vi "ECG_YY.vi"() -> ()   [LabVIEW 2020]
uses:
  <vilib>/Analysis/3filter.llb/Filter Passband Type.ctl
  <vilib>/Analysis/2dsp.llb/Real FFT.vi
  <vilib>/Utility/file.llb/Read Delimited Spreadsheet (DBL).vi
  <vilib>/Analysis/3filter.llb/Butterworth Filter (DBL).vi
  <vilib>/Analysis/NI_AALBase.lvlib
  <vilib>/Analysis/NI_AALPro.lvlib
panel:
  out "YY_stimuli4":dbl[](graph)
  out "YY_stimuli3":dbl[](graph)
  out "YY_stimuli1":dbl[](graph)
  out "YY_baseline":dbl[](graph)
  out "YY_stimuli 2":dbl[](graph)
  out "RRI_series_YY_baseline 2":dbl[](graph)
  out "PS_YY_stimuli4":cluster{"x":dbl, "x":dbl, dbl[]}(graph)
  out "PS_YY_stimuli 2":cluster{"x":dbl, "x":dbl, dbl[]}(graph)
  out "PS_YY_stimuli3":cluster{"x":dbl, "x":dbl, dbl[]}(graph)
  out "PS_YY_stimuli1":cluster{"x":dbl, "x":dbl, dbl[]}(graph)
  out "PS_YY_baseline":cluster{"x":dbl, "x":dbl, dbl[]}(graph)
  out "RRI_series_YY_stimuli4":dbl[](graph)
  out "RRI_series_YY_stimuli3":dbl[](graph)
  out "RRI_series_YY_stimuli2":dbl[](graph)
  out "RRI_series_YY_stimuli1":dbl[](graph)
  out "RRI_series_YY_baseline":dbl[](graph)
  out "YY_stimuli4":dbl[](graph)
  out "YY_stimuli3":dbl[](graph)
  out "YY_stimuli 2":dbl[](graph)
  out "YY_stimuli1":dbl[](graph)
  out "YY_baseline":dbl[](graph)
  out "psd_size 5":i32
  out "PS_WD_stimuli4":cluster{"x":dbl, "x":dbl, dbl[]}(graph)
  out "LF/HF 5":dbl
  out "HF  2":dbl
  out "LF  2":dbl
  out "TP (<=0.4Hz)  2":dbl
  out "RRI_size 5":i32
  out "RRI_series_YY_stimuli4":dbl[](graph)
  out "RRI series 5":dbl[](array[numeric])
  out "size(s) 5":i32
  out "2nd Derivatives 5":dbl[](array[numeric])
  out "Amplitudes 5":dbl[](array[numeric])
  out "amplitude 5":dbl[](array[numeric])
  out "location 5":dbl[](array[numeric])
  out "Locations 5":dbl[](array[numeric])
  in  "file path (dialog if empty) 5":path
  out "psd_size 4":i32
  out "PS_WD_stimuli3":cluster{"x":dbl, "x":dbl, dbl[]}(graph)
  out "LF/HF 4":dbl
  out "HF  2":dbl
  out "LF  2":dbl
  out "TP (<=0.4Hz)  2":dbl
  out "RRI_size 4":i32
  out "RRI_series_YY_stimuli3":dbl[](graph)
  out "RRI series 4":dbl[](array[numeric])
  out "size(s) 4":i32
  out "2nd Derivatives 4":dbl[](array[numeric])
  out "Amplitudes 4":dbl[](array[numeric])
  out "amplitude 4":dbl[](array[numeric])
  out "location 4":dbl[](array[numeric])
  out "Locations 4":dbl[](array[numeric])
  in  "file path (dialog if empty) 4":path
  out "psd_size 3":i32
  out "PS_WD_stimuli 2":cluster{"x":dbl, "x":dbl, dbl[]}(graph)
  out "LF/HF 3":dbl
  out "HF  2":dbl
  out "LF  2":dbl
  out "TP (<=0.4Hz)  2":dbl
  out "RRI_size 3":i32
  out "RRI_series_YY_stimuli2":dbl[](graph)
  out "RRI series 3":dbl[](array[numeric])
  out "size(s) 3":i32
  out "2nd Derivatives 3":dbl[](array[numeric])
  out "Amplitudes 3":dbl[](array[numeric])
  out "amplitude 3":dbl[](array[numeric])
  out "location 3":dbl[](array[numeric])
  out "Locations 3":dbl[](array[numeric])
  in  "file path (dialog if empty) 3":path
  out "psd_size 2":i32
  out "PS_WD_stimuli1":cluster{"x":dbl, "x":dbl, dbl[]}(graph)
  out "LF/HF 2":dbl
  out "HF  2":dbl
  out "LF  2":dbl
  out "TP (<=0.4Hz)  2":dbl
  out "RRI_size 2":i32
  out "RRI_series_YY_stimuli1":dbl[](graph)
  out "RRI series 2":dbl[](array[numeric])
  out "size(s) 2":i32
  out "2nd Derivatives 2":dbl[](array[numeric])
  out "Amplitudes 2":dbl[](array[numeric])
  out "amplitude 2":dbl[](array[numeric])
  out "location 2":dbl[](array[numeric])
  out "Locations 2":dbl[](array[numeric])
  in  "file path (dialog if empty) 2":path
  out "psd_size":i32
  out "PS_WD_baseline":cluster{"x":dbl, "x":dbl, dbl[]}(graph)
  out "LF/HF":dbl
  out "HF":dbl
  out "LF":dbl
  out "TP (<=0.4Hz)":dbl
  out "RRI_size":i32
  out "RRI_series_YY_baseline":dbl[](graph)
  out "RRI series":dbl[](array[numeric])
  out "size(s)":i32
  out "2nd Derivatives":dbl[](array[numeric])
  out "Amplitudes":dbl[](array[numeric])
  out "amplitude":dbl[](array[numeric])
  out "location":dbl[](array[numeric])
  out "Locations":dbl[](array[numeric])
  in  "file path (dialog if empty)":path
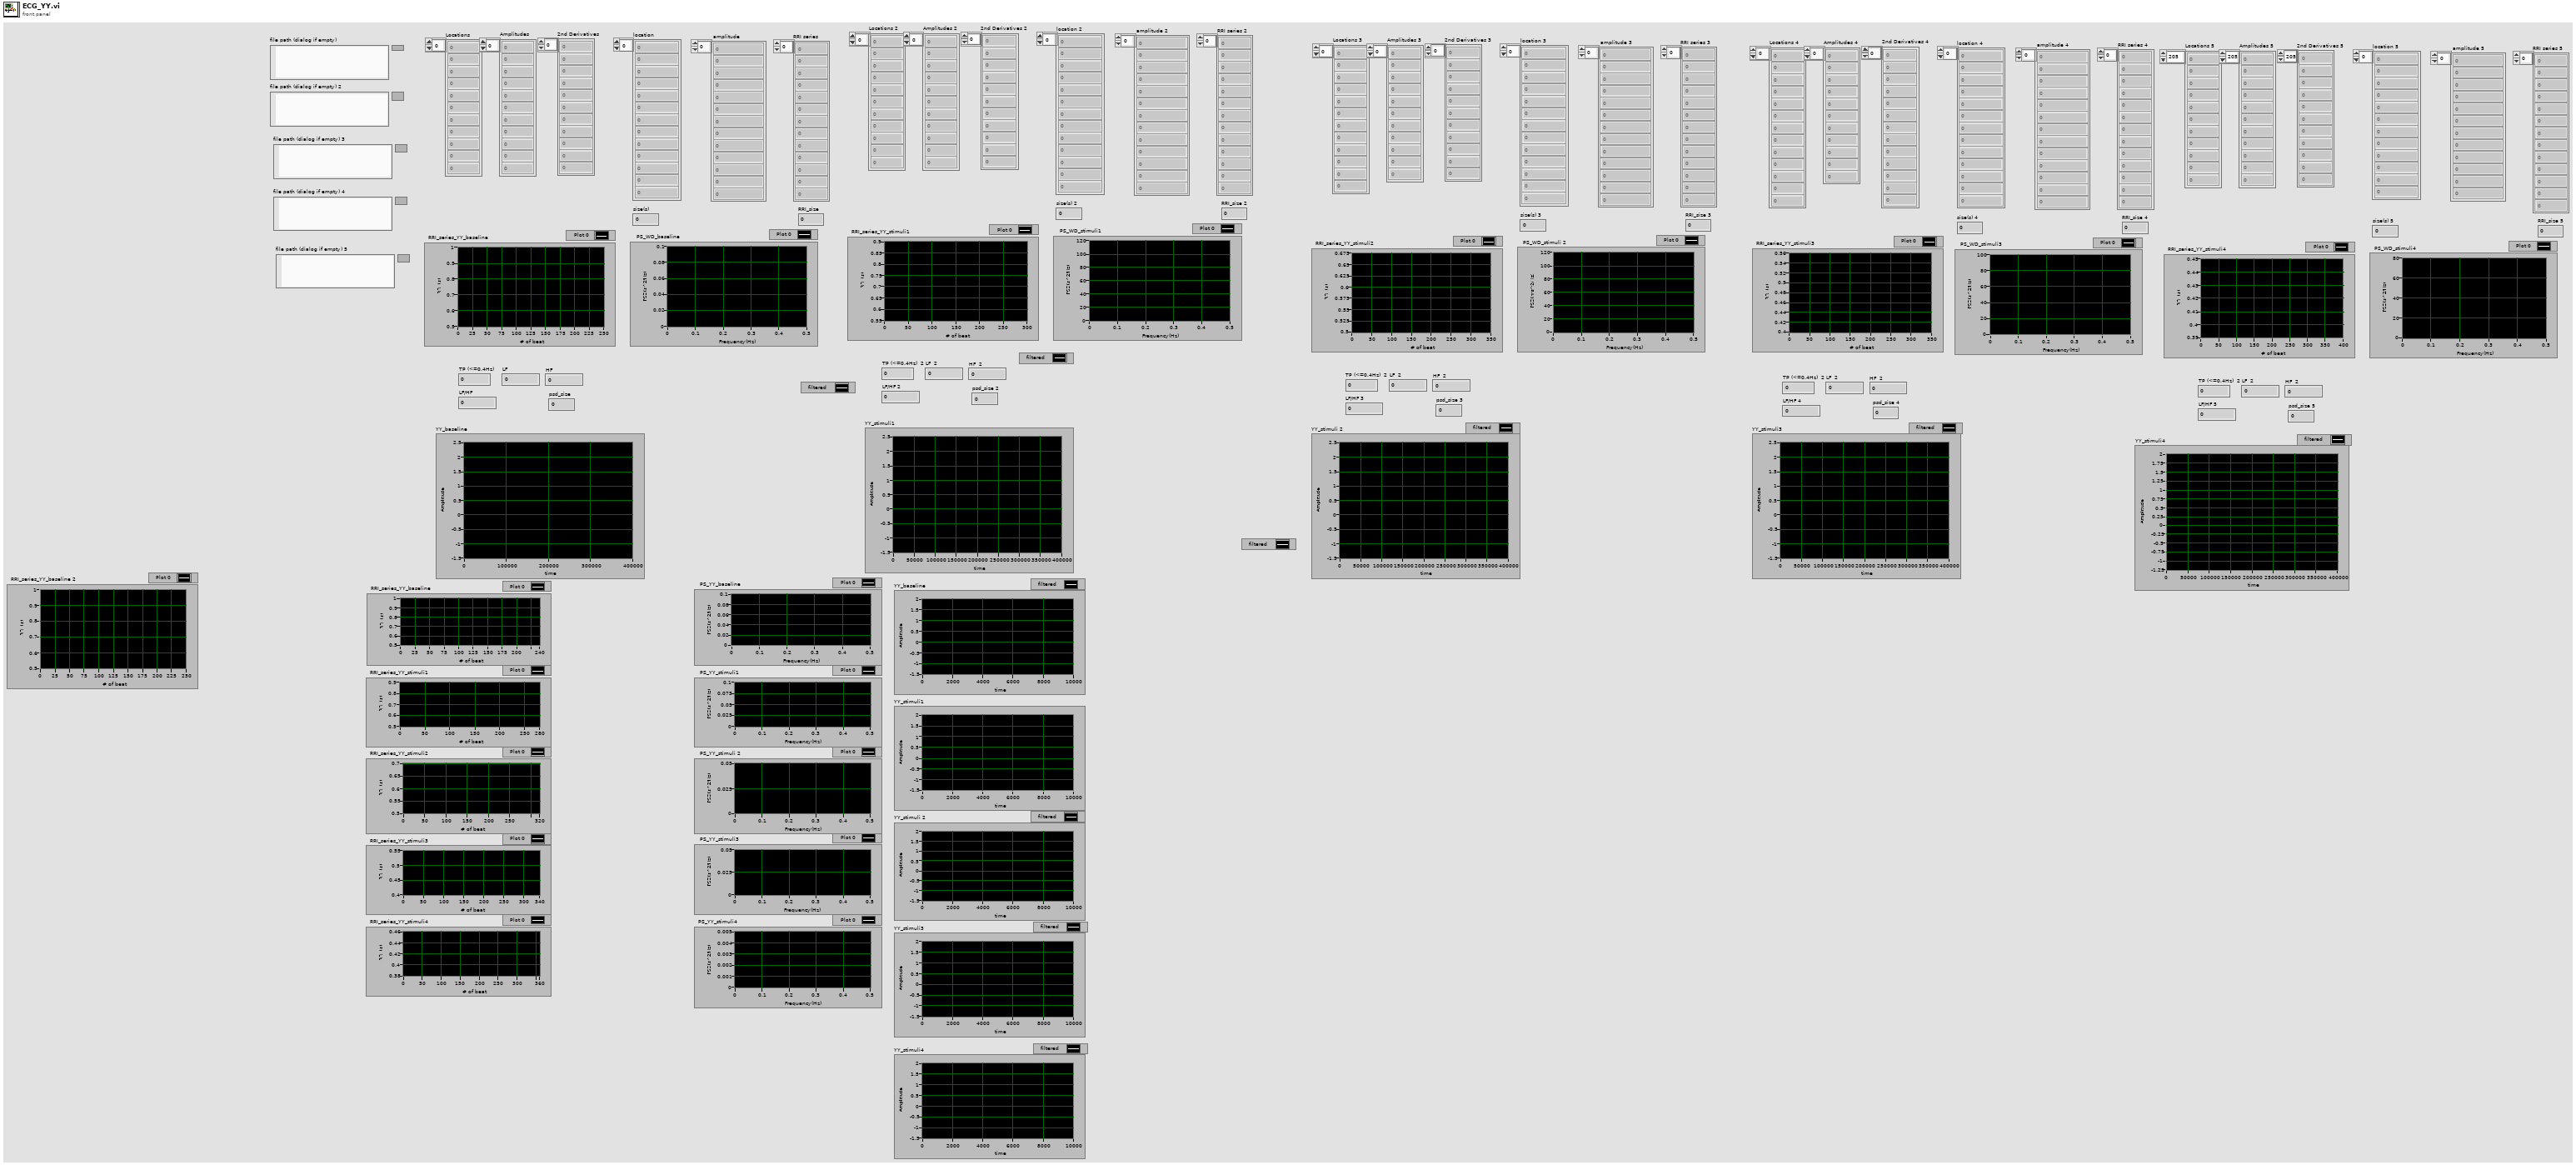
[diagram p1: front panel]
types:
  T1 = typedef "NI_AALBase.lvlib/Filter Passband Type.ctl" = enum32{"Lowpass", "Highpass", "Bandpass", "Bandstop"}
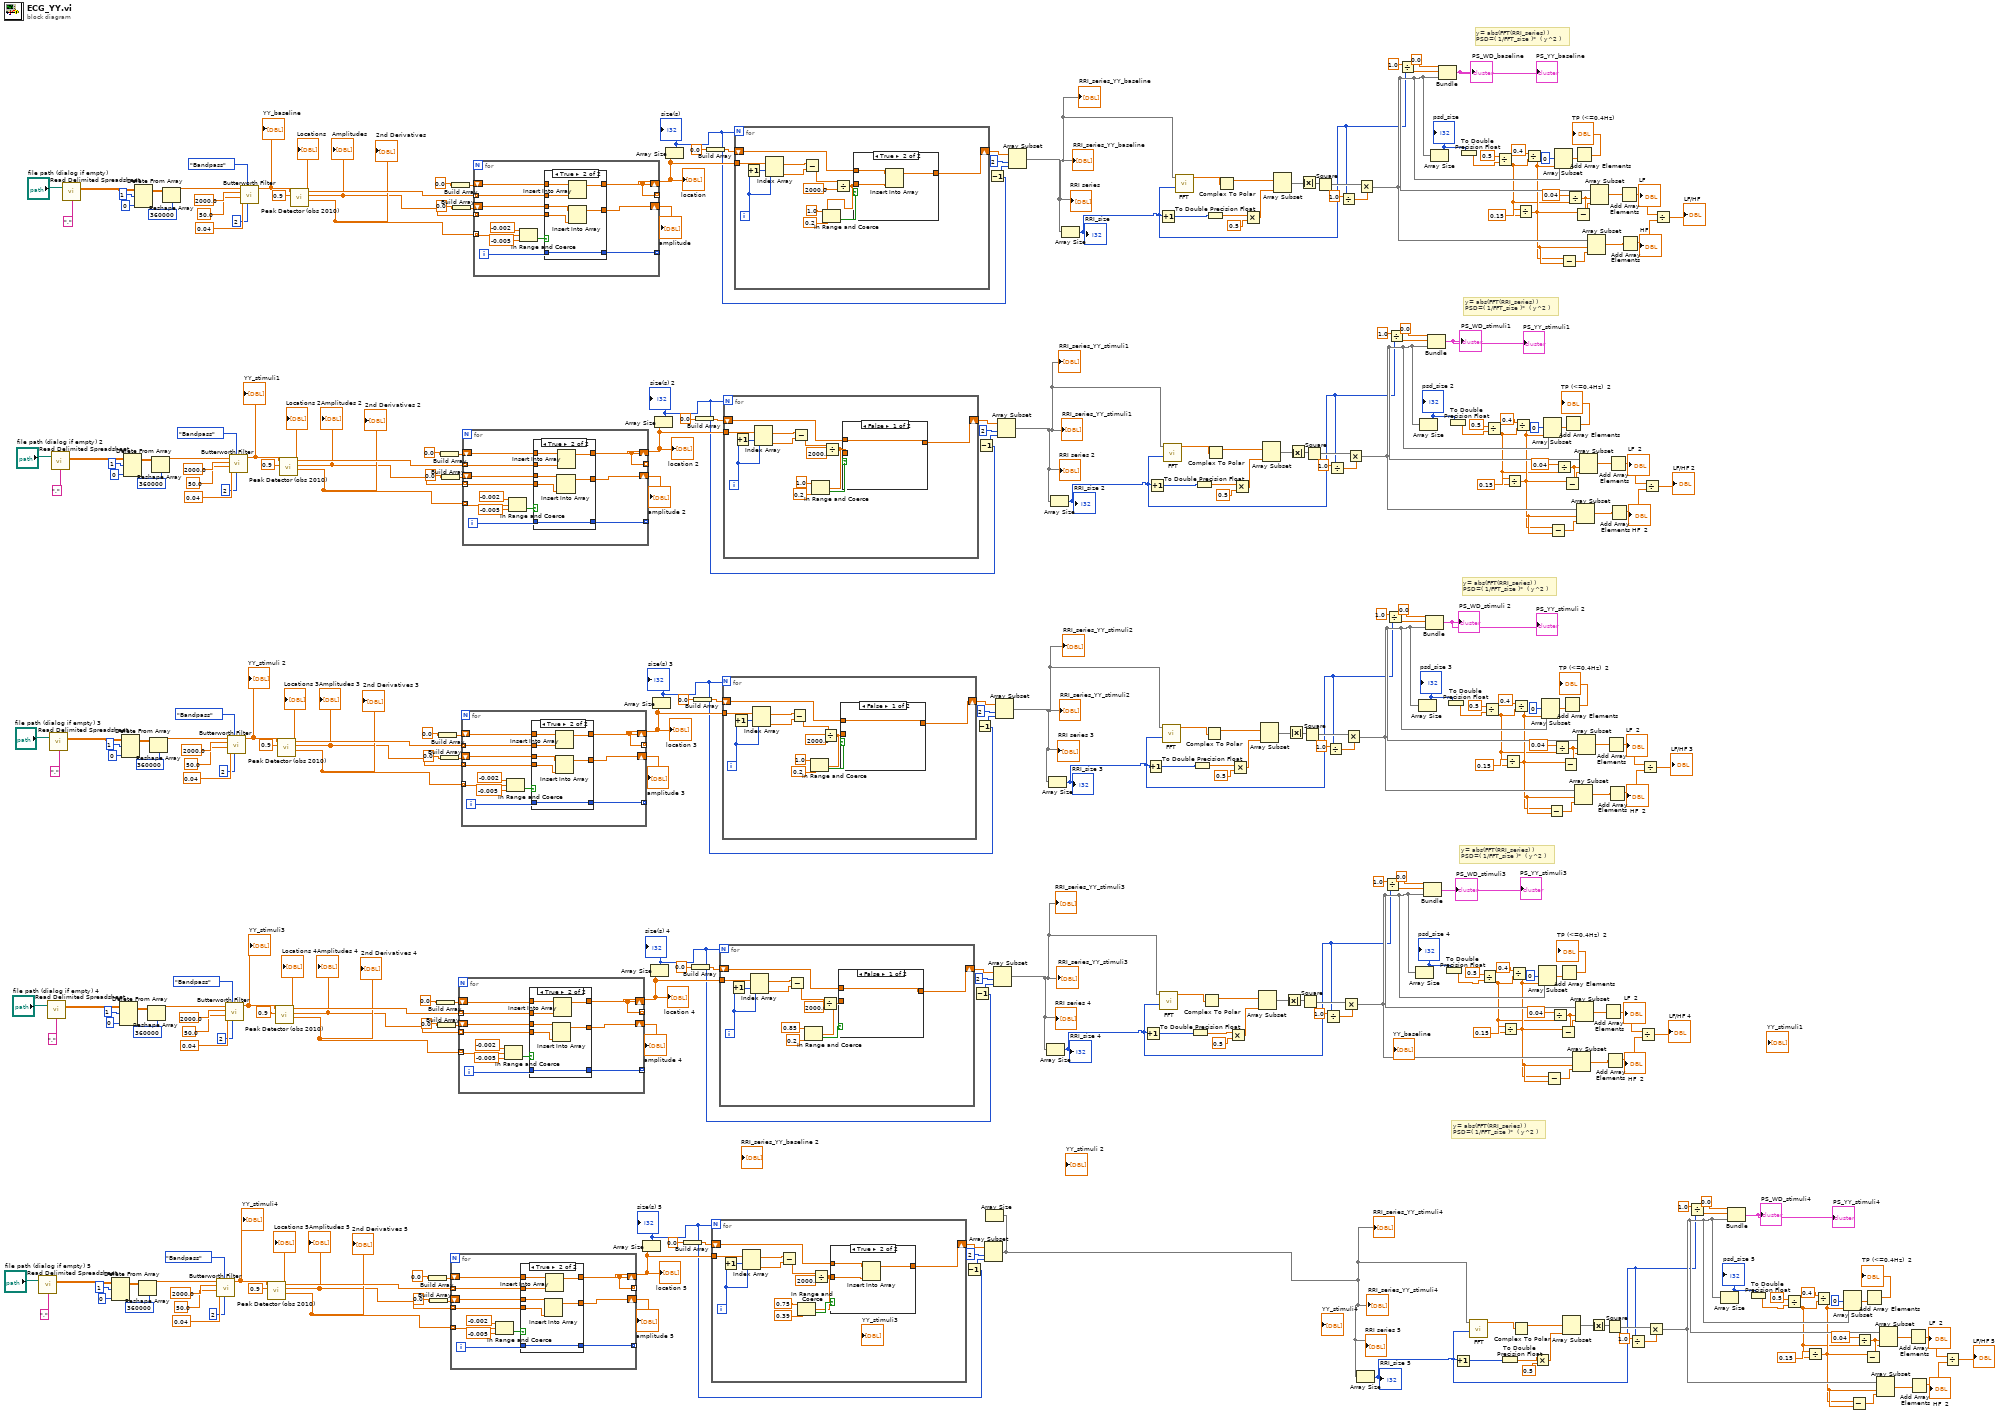
[diagram p0: block diagram]
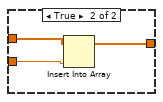
[diagram p4: hidden frame]
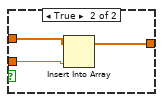
[diagram p6: hidden frame]
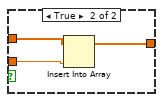
[diagram p8: hidden frame]
diagram:
  # "y= abs(FFT(RRI_series) )         \nPSD=( 1/FFT_size )*  ( y^2 )"
  # "y= abs(FFT(RRI_series) )         \nPSD=( 1/FFT_size )*  ( y^2 )"
  # "y= abs(FFT(RRI_series) )         \nPSD=( 1/FFT_size )*  ( y^2 )"
  # "y= abs(FFT(RRI_series) )         \nPSD=( 1/FFT_size )*  ( y^2 )"
  # "y= abs(FFT(RRI_series) )         \nPSD=( 1/FFT_size )*  ( y^2 )"
  n1 = call-poly <vilib>:"Read Delimited Spreadsheet.vi"("file path (dialog if empty)"="file path (dialog if empty) 5", "delimiter (\\t)"="," ("delimiter (\\t)")) -> ("all rows"=w79:dbl[][])  [unwired: 8 in, 5 out]
  n2 = call-poly <vilib>:"Read Delimited Spreadsheet.vi"("file path (dialog if empty)"="file path (dialog if empty) 4", "delimiter (\\t)"="," ("delimiter (\\t)")) -> ("all rows"=w144:dbl[][])  [unwired: 8 in, 5 out]
  n3 = call-poly <vilib>:"Read Delimited Spreadsheet.vi"("file path (dialog if empty)"="file path (dialog if empty) 3", "delimiter (\\t)"="," ("delimiter (\\t)")) -> ("all rows"=w209:dbl[][])  [unwired: 8 in, 5 out]
  n4 = call-poly <vilib>:"Read Delimited Spreadsheet.vi"("file path (dialog if empty)"="file path (dialog if empty) 2", "delimiter (\\t)"="," ("delimiter (\\t)")) -> ("all rows"=w274:dbl[][])  [unwired: 8 in, 5 out]
  n5 = call-poly <vilib>:"Read Delimited Spreadsheet.vi"("file path (dialog if empty)"="file path (dialog if empty)", "delimiter (\\t)"="," ("delimiter (\\t)")) -> ("all rows"=w339:dbl[][])  [unwired: 8 in, 5 out]
  n6 = Delete From Array(array=w79, length=1, index (col)=0 ("disabled index (col)")) -> (array with subset deleted=w69:dbl[][])  [unwired: 1 in, 1 out]
  n7 = Delete From Array(array=w144, length=1, index (col)=0 ("disabled index (col)")) -> (array with subset deleted=w134:dbl[][])  [unwired: 1 in, 1 out]
  n8 = Delete From Array(array=w209, length=1, index (col)=0 ("disabled index (col)")) -> (array with subset deleted=w199:dbl[][])  [unwired: 1 in, 1 out]
  n9 = Delete From Array(array=w274, length=1, index (col)=0 ("disabled index (col)")) -> (array with subset deleted=w264:dbl[][])  [unwired: 1 in, 1 out]
  n10 = Delete From Array(array=w339, length=1, index (col)=0 ("disabled index (col)")) -> (array with subset deleted=w329:dbl[][])  [unwired: 1 in, 1 out]
  n11 = Reshape Array(w69, 360000 ("dimension size")) -> (w68:dbl[])
  n12 = Reshape Array(w134, 360000 ("dimension size")) -> (w133:dbl[])
  n13 = Reshape Array(w199, 360000 ("dimension size")) -> (w198:dbl[])
  n14 = Reshape Array(w264, 360000 ("dimension size")) -> (w263:dbl[])
  n15 = Reshape Array(w329, 360000 ("dimension size")) -> (w328:dbl[])
  n16 = call-poly <vilib>:"Butterworth Filter.vi"("order"=2, "filter type"=Filter_Passband_Type."Bandpass", "low cutoff freq: fl"=0.04, "high cutoff freq: fh"=50.0, "sampling freq: fs"=2000.0, "X"=w68) -> ("Filtered X"=w12:dbl[])  [unwired: 2 in, 1 out]
  "YY_stimuli4" <- w12
  n17 = call-poly <vilib>:"Butterworth Filter.vi"("order"=2, "filter type"=Filter_Passband_Type."Bandpass", "low cutoff freq: fl"=0.04, "high cutoff freq: fh"=50.0, "sampling freq: fs"=2000.0, "X"=w133) -> ("Filtered X"=w13:dbl[])  [unwired: 2 in, 1 out]
  "YY_stimuli3" <- w13
  n18 = call-poly <vilib>:"Butterworth Filter.vi"("order"=2, "filter type"=Filter_Passband_Type."Bandpass", "low cutoff freq: fl"=0.04, "high cutoff freq: fh"=50.0, "sampling freq: fs"=2000.0, "X"=w198) -> ("Filtered X"=w14:dbl[])  [unwired: 2 in, 1 out]
  "YY_stimuli 2" <- w14
  n19 = call-poly <vilib>:"Butterworth Filter.vi"("order"=2, "filter type"=Filter_Passband_Type."Bandpass", "low cutoff freq: fl"=0.04, "high cutoff freq: fh"=50.0, "sampling freq: fs"=2000.0, "X"=w263) -> ("Filtered X"=w15:dbl[])  [unwired: 2 in, 1 out]
  "YY_stimuli1" <- w15
  n20 = call-poly <vilib>:"Butterworth Filter.vi"("order"=2, "filter type"=Filter_Passband_Type."Bandpass", "low cutoff freq: fl"=0.04, "high cutoff freq: fh"=50.0, "sampling freq: fs"=2000.0, "X"=w328) -> ("Filtered X"=w16:dbl[])  [unwired: 2 in, 1 out]
  "YY_baseline" <- w16
  n21 = call <vilib>:"Peak Detector (obs 2010).vi"("threshold"=0.9, "X"=w12) -> ("2nd Derivatives"=w62:dbl[], "Amplitudes"=w59:dbl[], "Locations"=w64:dbl[])  [unwired: 5 in, 2 out]
  "Locations 5" <- w64
  "Amplitudes 5" <- w59
  "2nd Derivatives 5" <- w62
  n22 = call <vilib>:"Peak Detector (obs 2010).vi"("threshold"=0.9, "X"=w13) -> ("2nd Derivatives"=w127:dbl[], "Amplitudes"=w124:dbl[], "Locations"=w129:dbl[])  [unwired: 5 in, 2 out]
  "Locations 4" <- w129
  "Amplitudes 4" <- w124
  "2nd Derivatives 4" <- w127
  n23 = call <vilib>:"Peak Detector (obs 2010).vi"("threshold"=0.9, "X"=w14) -> ("2nd Derivatives"=w192:dbl[], "Amplitudes"=w189:dbl[], "Locations"=w194:dbl[])  [unwired: 5 in, 2 out]
  "Locations 3" <- w194
  "Amplitudes 3" <- w189
  "2nd Derivatives 3" <- w192
  n24 = call <vilib>:"Peak Detector (obs 2010).vi"("threshold"=0.9, "X"=w15) -> ("2nd Derivatives"=w257:dbl[], "Amplitudes"=w254:dbl[], "Locations"=w259:dbl[])  [unwired: 5 in, 2 out]
  "Locations 2" <- w259
  "Amplitudes 2" <- w254
  "2nd Derivatives 2" <- w257
  n25 = call <vilib>:"Peak Detector (obs 2010).vi"("threshold"=0.9, "X"=w16) -> ("2nd Derivatives"=w322:dbl[], "Amplitudes"=w319:dbl[], "Locations"=w324:dbl[])  [unwired: 5 in, 2 out]
  "Locations" <- w324
  "Amplitudes" <- w319
  "2nd Derivatives" <- w322
  n26 = Build Array(0.0 ("element")) -> (w66:dbl[])
  n27 = Build Array(0.0 ("element")) -> (w60:dbl[])
  n28 = Build Array(0.0 ("element")) -> (w131:dbl[])
  n29 = Build Array(0.0 ("element")) -> (w125:dbl[])
  n30 = Build Array(0.0 ("element")) -> (w196:dbl[])
  n31 = Build Array(0.0 ("element")) -> (w190:dbl[])
  n32 = Build Array(0.0 ("element")) -> (w261:dbl[])
  n33 = Build Array(0.0 ("element")) -> (w255:dbl[])
  n34 = for {
    tunnel: w62 -> [w346] mode=indexing
    shift-right: [w341] -> w58
    shift-left: w66 -> [w349]
    tunnel: [w347] -> _ mode=indexing
    tunnel: w64 -> [w345] mode=indexing
    shift-right: [w343] -> w63
    shift-left: w60 -> [w344]
    tunnel: w59 -> [w342] mode=indexing
    tunnel: [w341] -> _ mode=indexing
    i -> [w348]
    n35 = In Range and Coerce(upper limit=-0.002, x=w346, lower limit=-0.005) -> (In Range?=w350:bool)  [unwired: 1 out]
    n36 = case shown="True" w350 {
      tunnel: w349 -> [w355 w362]
      tunnel: [w355 w361] -> w341
      tunnel: [w354 w360] -> w347
      tunnel: w348 -> [w354 w360]
      tunnel: w345 -> [_ w359]
      tunnel: w344 -> [w353 w358]
      tunnel: [w353 w357] -> w343
      tunnel: w342 -> [_ w356]
      frame False {
      }
      frame True {
        n37 = Insert Into Array(array=w358, new element=w356) -> (w357:dbl[])  [unwired: 1 in]
        n38 = Insert Into Array(array=w362, new element=w359) -> (w361:dbl[])  [unwired: 1 in]
      }
    }
  }
  "location 5" <- w58
  "amplitude 5" <- w63
  n39 = Build Array(0.0 ("element")) -> (w326:dbl[])
  n40 = Build Array(0.0 ("element")) -> (w320:dbl[])
  n41 = for {
    tunnel: w127 -> [w368] mode=indexing
    shift-right: [w363] -> w123
    shift-left: w131 -> [w371]
    tunnel: [w369] -> _ mode=indexing
    tunnel: w129 -> [w367] mode=indexing
    shift-right: [w365] -> w128
    shift-left: w125 -> [w366]
    tunnel: w124 -> [w364] mode=indexing
    tunnel: [w363] -> _ mode=indexing
    i -> [w370]
    n42 = In Range and Coerce(upper limit=-0.002, x=w368, lower limit=-0.005) -> (In Range?=w372:bool)  [unwired: 1 out]
    n43 = case shown="True" w372 {
      tunnel: w371 -> [w377 w384]
      tunnel: [w377 w383] -> w363
      tunnel: [w376 w382] -> w369
      tunnel: w370 -> [w376 w382]
      tunnel: w367 -> [_ w381]
      tunnel: w366 -> [w375 w380]
      tunnel: [w375 w379] -> w365
      tunnel: w364 -> [_ w378]
      frame False {
      }
      frame True {
        n44 = Insert Into Array(array=w380, new element=w378) -> (w379:dbl[])  [unwired: 1 in]
        n45 = Insert Into Array(array=w384, new element=w381) -> (w383:dbl[])  [unwired: 1 in]
      }
    }
  }
  "location 4" <- w123
  "amplitude 4" <- w128
  n46 = for {
    tunnel: w192 -> [w390] mode=indexing
    shift-right: [w385] -> w188
    shift-left: w196 -> [w393]
    tunnel: [w391] -> _ mode=indexing
    tunnel: w194 -> [w389] mode=indexing
    shift-right: [w387] -> w193
    shift-left: w190 -> [w388]
    tunnel: w189 -> [w386] mode=indexing
    tunnel: [w385] -> _ mode=indexing
    i -> [w392]
    n47 = In Range and Coerce(upper limit=-0.002, x=w390, lower limit=-0.005) -> (In Range?=w394:bool)  [unwired: 1 out]
    n48 = case shown="True" w394 {
      tunnel: w393 -> [w399 w406]
      tunnel: [w399 w405] -> w385
      tunnel: [w398 w404] -> w391
      tunnel: w392 -> [w398 w404]
      tunnel: w389 -> [_ w403]
      tunnel: w388 -> [w397 w402]
      tunnel: [w397 w401] -> w387
      tunnel: w386 -> [_ w400]
      frame False {
      }
      frame True {
        n49 = Insert Into Array(array=w402, new element=w400) -> (w401:dbl[])  [unwired: 1 in]
        n50 = Insert Into Array(array=w406, new element=w403) -> (w405:dbl[])  [unwired: 1 in]
      }
    }
  }
  "location 3" <- w188
  "amplitude 3" <- w193
  n51 = for {
    tunnel: w257 -> [w412] mode=indexing
    shift-right: [w407] -> w253
    shift-left: w261 -> [w415]
    tunnel: [w413] -> _ mode=indexing
    tunnel: w259 -> [w411] mode=indexing
    shift-right: [w409] -> w258
    shift-left: w255 -> [w410]
    tunnel: w254 -> [w408] mode=indexing
    tunnel: [w407] -> _ mode=indexing
    i -> [w414]
    n52 = In Range and Coerce(upper limit=-0.002, x=w412, lower limit=-0.005) -> (In Range?=w416:bool)  [unwired: 1 out]
    n53 = case shown="True" w416 {
      tunnel: w415 -> [w421 w428]
      tunnel: [w421 w427] -> w407
      tunnel: [w420 w426] -> w413
      tunnel: w414 -> [w420 w426]
      tunnel: w411 -> [_ w425]
      tunnel: w410 -> [w419 w424]
      tunnel: [w419 w423] -> w409
      tunnel: w408 -> [_ w422]
      frame False {
      }
      frame True {
        n54 = Insert Into Array(array=w424, new element=w422) -> (w423:dbl[])  [unwired: 1 in]
        n55 = Insert Into Array(array=w428, new element=w425) -> (w427:dbl[])  [unwired: 1 in]
      }
    }
  }
  "location 2" <- w253
  "amplitude 2" <- w258
  n56 = for {
    tunnel: w322 -> [w434] mode=indexing
    shift-right: [w429] -> w318
    shift-left: w326 -> [w437]
    tunnel: [w435] -> _ mode=indexing
    tunnel: w324 -> [w433] mode=indexing
    shift-right: [w431] -> w323
    shift-left: w320 -> [w432]
    tunnel: w319 -> [w430] mode=indexing
    tunnel: [w429] -> _ mode=indexing
    i -> [w436]
    n57 = In Range and Coerce(upper limit=-0.002, x=w434, lower limit=-0.005) -> (In Range?=w438:bool)  [unwired: 1 out]
    n58 = case shown="True" w438 {
      tunnel: w437 -> [w443 w450]
      tunnel: [w443 w449] -> w429
      tunnel: [w442 w448] -> w435
      tunnel: w436 -> [w442 w448]
      tunnel: w433 -> [_ w447]
      tunnel: w432 -> [w441 w446]
      tunnel: [w441 w445] -> w431
      tunnel: w430 -> [_ w444]
      frame False {
      }
      frame True {
        n59 = Insert Into Array(array=w446, new element=w444) -> (w445:dbl[])  [unwired: 1 in]
        n60 = Insert Into Array(array=w450, new element=w447) -> (w449:dbl[])  [unwired: 1 in]
      }
    }
  }
  "location" <- w318
  "amplitude" <- w323
  n61 = Array Size(array=w58) -> (size(s)=w54:i32)
  "size(s) 5" <- w54
  n62 = Array Size(array=w123) -> (size(s)=w118:i32)
  "size(s) 4" <- w118
  n63 = Array Size(array=w188) -> (size(s)=w183:i32)
  "size(s) 3" <- w183
  n64 = Array Size(array=w253) -> (size(s)=w248:i32)
  "size(s) 2" <- w248
  n65 = Array Size(array=w318) -> (size(s)=w313:i32)
  "size(s)" <- w313
  n66 = Build Array(0.0 ("array")) -> (w56:dbl[])
  n67 = Build Array(0.0 ("array")) -> (w121:dbl[])
  n68 = Build Array(0.0 ("array")) -> (w186:dbl[])
  n69 = Build Array(0.0 ("array")) -> (w251:dbl[])
  n70 = Build Array(0.0 ("array")) -> (w316:dbl[])
  n71 = for {
    N: w54 -> [_]
    tunnel: w58 -> [w460]
    shift-right: [w455] -> w3
    shift-left: w56 -> [w456]
    i -> [w462]
    n72 = Increment(x=w462) -> (x+1=w463:i32)
    n73 = Index Array(array=w460, index #1=w463, index #2=w462) -> (element #1=w461:dbl, element #2=w459:dbl)
    n74 = Subtract(x=w461, y=w459) -> (x-y=w452:dbl)
    n75 = Divide(x=w452, y=2000.0) -> (x/y=w451:dbl)
    n76 = In Range and Coerce(upper limit=0.75, x=w451, lower limit=0.39) -> (In Range?=w454:bool)  [unwired: 1 out]
    n77 = case shown="True" w454 {
      tunnel: w456 -> [w464 w467]
      tunnel: w451 -> [_ w466]
      tunnel: [w464 w465] -> w455
      frame False {
      }
      frame True {
        n78 = Insert Into Array(array=w467, new element=w466) -> (w465:dbl[])  [unwired: 1 in]
      }
    }
  }
  n79 = for {
    N: w118 -> [_]
    tunnel: w123 -> [w477]
    shift-right: [w471] -> w120
    shift-left: w121 -> [w472]
    i -> [w479]
    n80 = Increment(x=w479) -> (x+1=w480:i32)
    n81 = Index Array(array=w477, index #1=w480, index #2=w479) -> (element #1=w478:dbl, element #2=w476:dbl)
    n82 = Subtract(x=w478, y=w476) -> (x-y=w469:dbl)
    n83 = Divide(x=w469, y=2000.0) -> (x/y=w468:dbl)
    n84 = In Range and Coerce(upper limit=0.85, x=w468, lower limit=0.2) -> (In Range?=w473:bool)  [unwired: 1 out]
    n85 = case shown="False" w473 {
      tunnel: w472 -> [w481 w484]
      tunnel: w468 -> [_ w483]
      tunnel: [w481 w482] -> w471
      frame False {
      }
      frame True {
        n86 = Insert Into Array(array=w484, new element=w483) -> (w482:dbl[])  [unwired: 1 in]
      }
    }
  }
  n87 = for {
    N: w183 -> [_]
    tunnel: w188 -> [w494]
    shift-right: [w488] -> w185
    shift-left: w186 -> [w489]
    i -> [w496]
    n88 = Increment(x=w496) -> (x+1=w497:i32)
    n89 = Index Array(array=w494, index #1=w497, index #2=w496) -> (element #1=w495:dbl, element #2=w493:dbl)
    n90 = Subtract(x=w495, y=w493) -> (x-y=w486:dbl)
    n91 = Divide(x=w486, y=2000.0) -> (x/y=w485:dbl)
    n92 = In Range and Coerce(upper limit=1.0, x=w485, lower limit=0.2) -> (In Range?=w490:bool)  [unwired: 1 out]
    n93 = case shown="False" w490 {
      tunnel: w489 -> [w498 w501]
      tunnel: w485 -> [_ w500]
      tunnel: [w498 w499] -> w488
      frame False {
      }
      frame True {
        n94 = Insert Into Array(array=w501, new element=w500) -> (w499:dbl[])  [unwired: 1 in]
      }
    }
  }
  n95 = for {
    N: w248 -> [_]
    tunnel: w253 -> [w511]
    shift-right: [w505] -> w250
    shift-left: w251 -> [w506]
    i -> [w513]
    n96 = Increment(x=w513) -> (x+1=w514:i32)
    n97 = Index Array(array=w511, index #1=w514, index #2=w513) -> (element #1=w512:dbl, element #2=w510:dbl)
    n98 = Subtract(x=w512, y=w510) -> (x-y=w503:dbl)
    n99 = Divide(x=w503, y=2000.0) -> (x/y=w502:dbl)
    n100 = In Range and Coerce(upper limit=1.0, x=w502, lower limit=0.2) -> (In Range?=w507:bool)  [unwired: 1 out]
    n101 = case shown="False" w507 {
      tunnel: w506 -> [w515 w518]
      tunnel: w502 -> [_ w517]
      tunnel: [w515 w516] -> w505
      frame False {
      }
      frame True {
        n102 = Insert Into Array(array=w518, new element=w517) -> (w516:dbl[])  [unwired: 1 in]
      }
    }
  }
  n103 = for {
    N: w313 -> [_]
    tunnel: w318 -> [w528]
    shift-right: [w522] -> w315
    shift-left: w316 -> [w523]
    i -> [w530]
    n104 = Increment(x=w530) -> (x+1=w531:i32)
    n105 = Index Array(array=w528, index #1=w531, index #2=w530) -> (element #1=w529:dbl, element #2=w527:dbl)
    n106 = Subtract(x=w529, y=w527) -> (x-y=w521:dbl)
    n107 = Divide(x=w521, y=2000.0) -> (x/y=w519:dbl)
    n108 = In Range and Coerce(upper limit=1.0, x=w519, lower limit=0.2) -> (In Range?=w524:bool)  [unwired: 1 out]
    n109 = case shown="True" w524 {
      tunnel: w523 -> [w532 w535]
      tunnel: w519 -> [_ w534]
      tunnel: [w532 w533] -> w522
      frame False {
      }
      frame True {
        n110 = Insert Into Array(array=w535, new element=w534) -> (w533:dbl[])  [unwired: 1 in]
      }
    }
  }
  n111 = Decrement(x=w54) -> (x-1=w53:i32)
  n112 = Decrement(x=w118) -> (x-1=w117:i32)
  n113 = Decrement(x=w183) -> (x-1=w182:i32)
  n114 = Decrement(x=w248) -> (x-1=w247:i32)
  n115 = Array Subset(array=w3, index=2, length=w53) -> (w1:dbl[])
  "RRI series 5" <- w1
  "RRI_series_YY_stimuli4" <- w1
  "RRI_series_YY_stimuli4" <- w1
  n116 = Array Size(array=w1) -> ()  [unwired: 1 out]
  n117 = Decrement(x=w313) -> (x-1=w312:i32)
  n118 = Array Subset(array=w120, index=2, length=w117) -> (w9:dbl[])
  "RRI series 4" <- w9
  "RRI_series_YY_stimuli3" <- w9
  "RRI_series_YY_stimuli3" <- w9
  n119 = Array Subset(array=w185, index=2, length=w182) -> (w10:dbl[])
  "RRI series 3" <- w10
  "RRI_series_YY_stimuli2" <- w10
  "RRI_series_YY_stimuli2" <- w10
  n120 = Array Subset(array=w250, index=2, length=w247) -> (w11:dbl[])
  "RRI series 2" <- w11
  "RRI_series_YY_stimuli1" <- w11
  "RRI_series_YY_stimuli1" <- w11
  n121 = Array Subset(array=w315, index=2, length=w312) -> (w2:dbl[])
  "RRI series" <- w2
  "RRI_series_YY_baseline" <- w2
  "RRI_series_YY_baseline" <- w2
  n122 = Array Size(array=w9) -> (size(s)=w97:i32)
  "RRI_size 4" <- w97
  n123 = Array Size(array=w10) -> (size(s)=w162:i32)
  "RRI_size 3" <- w162
  n124 = Array Size(array=w11) -> (size(s)=w227:i32)
  "RRI_size 2" <- w227
  n125 = Array Size(array=w2) -> (size(s)=w292:i32)
  "RRI_size" <- w292
  n126 = Increment(x=w97) -> (x+1=w116:i32)
  n127 = Increment(x=w162) -> (x+1=w181:i32)
  n128 = Increment(x=w227) -> (x+1=w246:i32)
  n129 = Increment(x=w292) -> (x+1=w311:i32)
  n130 = call-poly <vilib>:"FFT.vi"("FFT size"=w97, "X"=w9) -> ("FFT {X}"=w96:cdb[])  [unwired: 8 in, 1 out]
  n131 = call-poly <vilib>:"FFT.vi"("FFT size"=w162, "X"=w10) -> ("FFT {X}"=w161:cdb[])  [unwired: 8 in, 1 out]
  n132 = call-poly <vilib>:"FFT.vi"("FFT size"=w227, "X"=w11) -> ("FFT {X}"=w226:cdb[])  [unwired: 8 in, 1 out]
  n133 = call-poly <vilib>:"FFT.vi"("FFT size"=w292, "X"=w2) -> ("FFT {X}"=w291:cdb[])  [unwired: 8 in, 1 out]
  n134 = To Double Precision Float(number=w116) -> (double precision float=w112:dbl)
  n135 = To Double Precision Float(number=w181) -> (double precision float=w177:dbl)
  n136 = To Double Precision Float(number=w246) -> (double precision float=w242:dbl)
  n137 = Complex To Polar(r * e^(i*theta)=w96) -> (r=w111:dbl[])  [unwired: 1 out]
  n138 = Complex To Polar(r * e^(i*theta)=w161) -> (r=w176:dbl[])  [unwired: 1 out]
  n139 = To Double Precision Float(number=w311) -> (double precision float=w307:dbl)
  n140 = Complex To Polar(r * e^(i*theta)=w226) -> (r=w241:dbl[])  [unwired: 1 out]
  n141 = Complex To Polar(r * e^(i*theta)=w291) -> (r=w306:dbl[])  [unwired: 1 out]
  n142 = Multiply(x=w112, y=0.5) -> (x*y=w114:dbl)
  n143 = Multiply(x=w177, y=0.5) -> (x*y=w179:dbl)
  n144 = Multiply(x=w242, y=0.5) -> (x*y=w244:dbl)
  n145 = Multiply(x=w307, y=0.5) -> (x*y=w309:dbl)
  n146 = Array Subset(array=w111, length=w114) -> (w102:dbl[])  [unwired: 1 in]
  n147 = Array Subset(array=w176, length=w179) -> (w167:dbl[])  [unwired: 1 in]
  n148 = Array Subset(array=w241, length=w244) -> (w232:dbl[])  [unwired: 1 in]
  n149 = Array Subset(array=w306, length=w309) -> (w297:dbl[])  [unwired: 1 in]
  n150 = Absolute Value(x=w102) -> (abs(x)=w101:dbl[])
  n151 = Absolute Value(x=w167) -> (abs(x)=w166:dbl[])
  n152 = Absolute Value(x=w232) -> (abs(x)=w231:dbl[])
  n153 = Absolute Value(x=w297) -> (abs(x)=w296:dbl[])
  n154 = Square(x=w101) -> (x^2=w100:dbl[])
  n155 = Square(x=w166) -> (x^2=w165:dbl[])
  n156 = Square(x=w231) -> (x^2=w230:dbl[])
  n157 = Square(x=w296) -> (x^2=w295:dbl[])
  n158 = Divide(x=1.0, y=w97) -> (x/y=w99:dbl)
  n159 = Divide(x=1.0, y=w162) -> (x/y=w164:dbl)
  n160 = Divide(x=1.0, y=w227) -> (x/y=w229:dbl)
  n161 = Divide(x=1.0, y=w292) -> (x/y=w294:dbl)
  n162 = Multiply(x=w100, y=w99) -> (x*y=w98:dbl[])
  n163 = Multiply(x=w165, y=w164) -> (x*y=w163:dbl[])
  n164 = Multiply(x=w230, y=w229) -> (x*y=w228:dbl[])
  n165 = Array Size(array=w1) -> (size(s)=w33:i32)
  "RRI_size 5" <- w33
  n166 = Multiply(x=w295, y=w294) -> (x*y=w293:dbl[])
  n167 = Divide(x=1.0, y=w97) -> (x/y=w103:dbl)
  n168 = Divide(x=1.0, y=w162) -> (x/y=w168:dbl)
  n169 = Divide(x=1.0, y=w227) -> (x/y=w233:dbl)
  n170 = Divide(x=1.0, y=w292) -> (x/y=w298:dbl)
  n171 = Array Size(array=w98) -> (size(s)=w95:i32)
  "psd_size 4" <- w95
  n172 = Array Size(array=w163) -> (size(s)=w160:i32)
  "psd_size 3" <- w160
  n173 = Array Size(array=w228) -> (size(s)=w225:i32)
  "psd_size 2" <- w225
  n174 = Bundle("x"=0.0, w103, w98) -> (→"PS_WD_stimuli3" →"PS_YY_stimuli3":cluster{"x":dbl, dbl, dbl[]})  [unwired: 1 in]
  n175 = Bundle("x"=0.0, w168, w163) -> (→"PS_WD_stimuli 2" →"PS_YY_stimuli 2":cluster{"x":dbl, dbl, dbl[]})  [unwired: 1 in]
  n176 = Bundle("x"=0.0, w233, w228) -> (→"PS_WD_stimuli1" →"PS_YY_stimuli1":cluster{"x":dbl, dbl, dbl[]})  [unwired: 1 in]
  n177 = Array Size(array=w293) -> (size(s)=w290:i32)
  "psd_size" <- w290
  n178 = Bundle("x"=0.0, w298, w293) -> (→"PS_WD_baseline" →"PS_YY_baseline":cluster{"x":dbl, dbl, dbl[]})  [unwired: 1 in]
  n179 = To Double Precision Float(number=w95) -> (double precision float=w84:dbl)
  n180 = To Double Precision Float(number=w160) -> (double precision float=w149:dbl)
  n181 = To Double Precision Float(number=w225) -> (double precision float=w214:dbl)
  n182 = Increment(x=w33) -> (x+1=w52:i32)
  n183 = To Double Precision Float(number=w290) -> (double precision float=w279:dbl)
  n184 = call-poly <vilib>:"FFT.vi"("FFT size"=w33, "X"=w1) -> ("FFT {X}"=w32:cdb[])  [unwired: 8 in, 1 out]
  n185 = Divide(x=0.5, y=w84) -> (x/y=w82:dbl)
  n186 = Divide(x=0.5, y=w149) -> (x/y=w147:dbl)
  n187 = Divide(x=0.5, y=w214) -> (x/y=w212:dbl)
  n188 = Divide(x=0.5, y=w279) -> (x/y=w277:dbl)
  n189 = To Double Precision Float(number=w52) -> (double precision float=w48:dbl)
  n190 = Divide(x=0.15, y=w82) -> (x/y=w88:dbl)
  n191 = Divide(x=0.15, y=w147) -> (x/y=w153:dbl)
  n192 = Divide(x=0.15, y=w212) -> (x/y=w218:dbl)
  n193 = Divide(x=0.4, y=w82) -> (x/y=w85:dbl)
  n194 = Divide(x=0.4, y=w147) -> (x/y=w150:dbl)
  n195 = Complex To Polar(r * e^(i*theta)=w32) -> (r=w47:dbl[])  [unwired: 1 out]
  n196 = Divide(x=0.4, y=w212) -> (x/y=w215:dbl)
  n197 = Divide(x=0.15, y=w277) -> (x/y=w283:dbl)
  n198 = Divide(x=0.4, y=w277) -> (x/y=w280:dbl)
  n199 = Multiply(x=w48, y=0.5) -> (x*y=w50:dbl)
  n200 = Array Subset(array=w98, index=0, length=w85) -> (w110:dbl[])
  n201 = Array Subset(array=w163, index=0, length=w150) -> (w175:dbl[])
  n202 = Array Subset(array=w228, index=0, length=w215) -> (w240:dbl[])
  n203 = Subtract(x=w85, y=w88) -> (x-y=w89:dbl)
  n204 = Subtract(x=w150, y=w153) -> (x-y=w154:dbl)
  n205 = Subtract(x=w215, y=w218) -> (x-y=w219:dbl)
  n206 = Divide(x=0.04, y=w82) -> (x/y=w91:dbl)
  n207 = Divide(x=0.04, y=w147) -> (x/y=w156:dbl)
  n208 = Array Subset(array=w293, index=0, length=w280) -> (w305:dbl[])
  n209 = Divide(x=0.04, y=w212) -> (x/y=w221:dbl)
  n210 = Subtract(x=w88, y=w91) -> (x-y=w90:dbl)
  n211 = Subtract(x=w280, y=w283) -> (x-y=w284:dbl)
  n212 = Add Array Elements(numeric array=w110) -> (sum=→"TP (<=0.4Hz)  2":dbl)
  n213 = Subtract(x=w153, y=w156) -> (x-y=w155:dbl)
  n214 = Add Array Elements(numeric array=w175) -> (sum=→"TP (<=0.4Hz)  2":dbl)
  n215 = Array Subset(array=w47, length=w50) -> (w38:dbl[])  [unwired: 1 in]
  n216 = Subtract(x=w218, y=w221) -> (x-y=w220:dbl)
  n217 = Add Array Elements(numeric array=w240) -> (sum=→"TP (<=0.4Hz)  2":dbl)
  n218 = Divide(x=0.04, y=w277) -> (x/y=w286:dbl)
  n219 = Array Subset(array=w98, index=w88, length=w89) -> (w86:dbl[])
  n220 = Subtract(x=w283, y=w286) -> (x-y=w285:dbl)
  n221 = Array Subset(array=w163, index=w153, length=w154) -> (w151:dbl[])
  n222 = Array Subset(array=w98, index=w91, length=w90) -> (w87:dbl[])
  n223 = Add Array Elements(numeric array=w305) -> (sum=→"TP (<=0.4Hz)":dbl)
  n224 = Array Subset(array=w228, index=w218, length=w219) -> (w216:dbl[])
  n225 = Array Subset(array=w163, index=w156, length=w155) -> (w152:dbl[])
  n226 = Array Subset(array=w228, index=w221, length=w220) -> (w217:dbl[])
  n227 = Array Subset(array=w293, index=w283, length=w284) -> (w281:dbl[])
  n228 = Absolute Value(x=w38) -> (abs(x)=w37:dbl[])
  n229 = Array Subset(array=w293, index=w286, length=w285) -> (w282:dbl[])
  n230 = Add Array Elements(numeric array=w87) -> (sum=w107:dbl)
  "LF  2" <- w107
  n231 = Add Array Elements(numeric array=w86) -> (sum=w106:dbl)
  "HF  2" <- w106
  n232 = Square(x=w37) -> (x^2=w36:dbl[])
  n233 = Add Array Elements(numeric array=w152) -> (sum=w172:dbl)
  "LF  2" <- w172
  n234 = Add Array Elements(numeric array=w151) -> (sum=w171:dbl)
  "HF  2" <- w171
  n235 = Add Array Elements(numeric array=w217) -> (sum=w237:dbl)
  "LF  2" <- w237
  n236 = Add Array Elements(numeric array=w216) -> (sum=w236:dbl)
  "HF  2" <- w236
  n237 = Add Array Elements(numeric array=w282) -> (sum=w302:dbl)
  "LF" <- w302
  n238 = Add Array Elements(numeric array=w281) -> (sum=w301:dbl)
  "HF" <- w301
  n239 = Divide(x=1.0, y=w33) -> (x/y=w35:dbl)
  n240 = Divide(x=w107, y=w106) -> (x/y=→"LF/HF 4":dbl)
  n241 = Divide(x=w172, y=w171) -> (x/y=→"LF/HF 3":dbl)
  n242 = Divide(x=w237, y=w236) -> (x/y=→"LF/HF 2":dbl)
  n243 = Multiply(x=w36, y=w35) -> (x*y=w34:dbl[])
  n244 = Divide(x=w302, y=w301) -> (x/y=→"LF/HF":dbl)
  n245 = Divide(x=1.0, y=w33) -> (x/y=w39:dbl)
  n246 = Array Size(array=w34) -> (size(s)=w31:i32)
  "psd_size 5" <- w31
  n247 = Bundle("x"=0.0, w39, w34) -> (→"PS_WD_stimuli4" →"PS_YY_stimuli4":cluster{"x":dbl, dbl, dbl[]})  [unwired: 1 in]
  n248 = To Double Precision Float(number=w31) -> (double precision float=w20:dbl)
  n249 = Divide(x=0.5, y=w20) -> (x/y=w18:dbl)
  n250 = Divide(x=0.15, y=w18) -> (x/y=w24:dbl)
  n251 = Divide(x=0.4, y=w18) -> (x/y=w21:dbl)
  n252 = Array Subset(array=w34, index=0, length=w21) -> (w46:dbl[])
  n253 = Subtract(x=w21, y=w24) -> (x-y=w25:dbl)
  n254 = Divide(x=0.04, y=w18) -> (x/y=w27:dbl)
  n255 = Subtract(x=w24, y=w27) -> (x-y=w26:dbl)
  n256 = Add Array Elements(numeric array=w46) -> (sum=→"TP (<=0.4Hz)  2":dbl)
  n257 = Array Subset(array=w34, index=w24, length=w25) -> (w22:dbl[])
  n258 = Array Subset(array=w34, index=w27, length=w26) -> (w23:dbl[])
  n259 = Add Array Elements(numeric array=w23) -> (sum=w43:dbl)
  "LF  2" <- w43
  n260 = Add Array Elements(numeric array=w22) -> (sum=w42:dbl)
  "HF  2" <- w42
  n261 = Divide(x=w43, y=w42) -> (x/y=→"LF/HF 5":dbl)
